vi "test.vi"() -> ()   [LabVIEW 2025]
uses:
  mydll.dll
panel:
  out "Numeric":i32
  in  "B":i32
  in  "A":i32
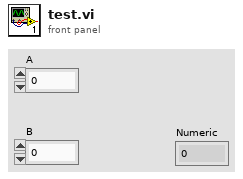
[diagram p1: front panel]
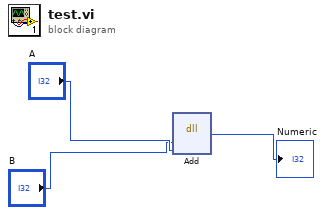
[diagram p0: block diagram]
diagram:
  n1 = dll-call lib="Z:/lab/workspace_window/labview-dll-template/mydll.dll" fn="Add"("a"="B", "b"="A") -> ("return"=→"Numeric":i32)  [unwired: 5 in, 2 out]
